vi "GEOM_File2keys.vi"(8 "error in (no error)":errorcluster, 10 "template in":string, 11 "ref dir":path) -> (0 "error out":errorcluster, 1 "header template":path, 2 "number of keywords found":i32, 3 "HeaderModules":T1[](array[typedef]))   [LabVIEW 2016]
doc: "This VI reads the configuration file searching for the \"infofile\" keyword. Then, it goes and reads the specified file, which should be a template for the TCS info format"
uses:
  GEOM_HeaderModule.ctl
panel:
  in  "HeaderModule":T1
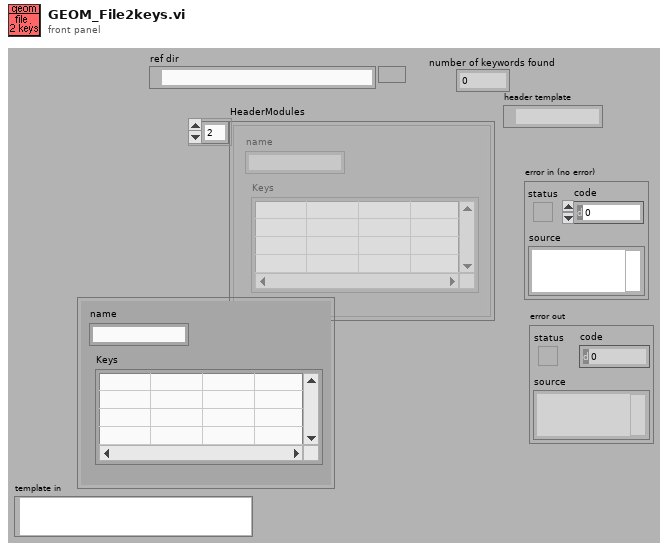
[diagram p1: front panel]
types:
  T1 = typedef "GEOM_HeaderModule.ctl" = cluster{"name":string, "Keys":string[][]}
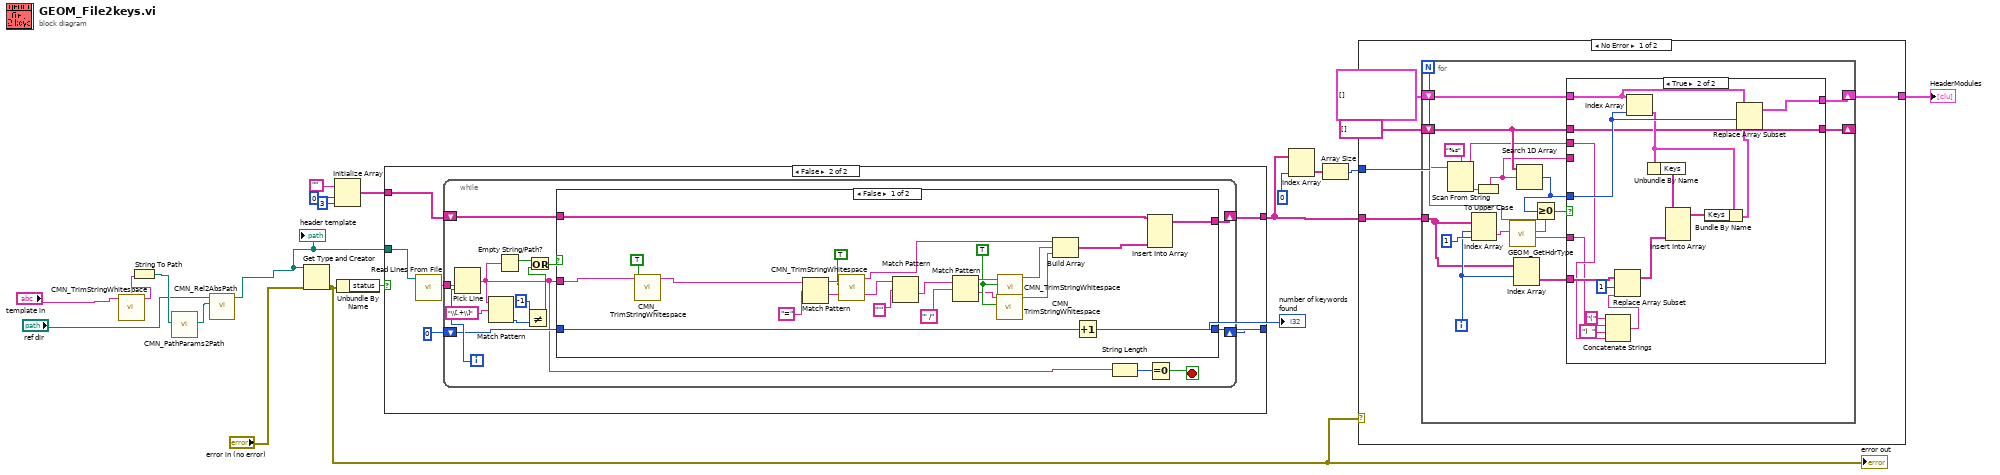
[diagram p0: block diagram]
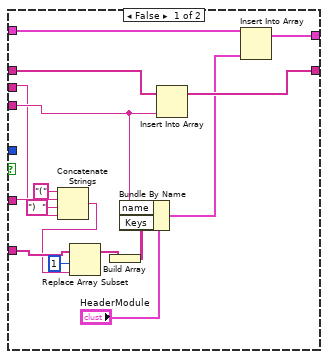
[diagram p2: hidden frame]
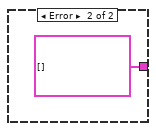
[diagram p3: hidden frame]
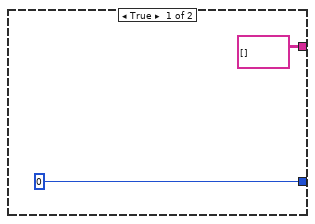
[diagram p4: hidden frame]
diagram:
  n1 = call "CMN_TrimStringWhitespace.vi"("string"="template in") -> ("trimmed string"=w5:string)  [unwired: 1 in, 8 out]
  n2 = String To Path(string=w5) -> (path=w4:path)
  n3 = call "CMN_PathParams2Path.vi"("Path In"=w4) -> ("Path out"=w3:path)  [unwired: 2 in, 8 out]
  n4 = call "CMN_Rel2AbsPath.vi"("test path"=w3, "absolute path"="ref dir") -> ("output path"=w13:path)  [unwired: 1 in, 8 out]
  "header template" <- w13
  n5 = Get Type and Creator(4:"error in (no error)", 7:w13) -> (0:w7:errorcluster)  [unwired: 3 out]
  "error out" <- w7
  n6 = Initialize Array("", 0, 3 ("dimension size")) -> (w15:string[][])
  n7 = Unbundle By Name(w7) -> ("status"=w18:bool)
  n8 = case shown="False" w18 {
    tunnel: w13 -> [_ w26]
    tunnel: [0 w23] -> w19
    tunnel: [string[][] [] w22] -> w11
    tunnel: w15 -> [_ w25]
    frame True {
    }
    frame False {
      n9 = call <vilib>:"Read Lines From File.vi"("file path (dialog if empty)"=w26) -> ("line string"=w27:string)  [unwired: 1 in, 7 out]
      n10 = while {
        shift-left: 0 -> [w32]
        shift-right: [w34] -> w23
        shift-left: w25 -> [w39]
        shift-right: [w38] -> w22
        tunnel: w27 -> [w42]
        i -> [w33]
        stop <- w40 stop-if-true
        n11 = Pick Line(multi-line string=w42, line index=w33) -> (output string=w29:string)  [unwired: 1 out]
        n12 = Match Pattern(string=w29, regular expression="\\[.+\\]") -> (offset past match=w36:i32)  [unwired: 4 out]
        n13 = Empty String/Path?(string/path=w29) -> (empty?=w31:bool)
        n14 = Not Equal?(x=-1, y=w36) -> (x != y?=w30:bool)
        n15 = Or(x=w31, y=w30) -> (x .or. y?=w28:bool)
        n16 = case shown="False" w28 {
          tunnel: w32 -> [w46 w64]
          tunnel: w39 -> [w50 w65]
          tunnel: [w49 w65] -> w38
          tunnel: [w45 w64] -> w34
          tunnel: w29 -> [w44 _]
          frame False {
            w55 = TRUE ("Both Ends?(F)")
            n17 = call "CMN_TrimStringWhitespace.vi"("Both Ends?(T)"=TRUE ("Both Ends?(F)"), "string"=w44) -> ("trimmed string"=w43:string)  [unwired: 8 out]
            n18 = Match Pattern(string=w43, regular expression="=") -> (before substring=w62:string, after substring=w61:string)  [unwired: 3 out]
            n19 = call "CMN_TrimStringWhitespace.vi"("Both Ends?(T)"=TRUE ("Both Ends?(F)"), "string"=w62) -> ("trimmed string"=w47:string)  [unwired: 8 out]
            n20 = Match Pattern(string=w61, regular expression="'") -> (after substring=w59:string)  [unwired: 4 out]
            n21 = Match Pattern(string=w59, regular expression="' /") -> (before substring=w57:string, after substring=w54:string)  [unwired: 3 out]
            n22 = call "CMN_TrimStringWhitespace.vi"("Both Ends?(T)"=w55, "string"=w54) -> ("trimmed string"=w52:string)  [unwired: 8 out]
            n23 = call "CMN_TrimStringWhitespace.vi"("Both Ends?(T)"=w55, "string"=w57) -> ("trimmed string"=w53:string)  [unwired: 8 out]
            n24 = Build Array(w47, w53, w52) -> (w51:string[])
            n25 = Increment(x=w46) -> (x+1=w45:i32)
            n26 = Insert Into Array(array=w50, new element=w51) -> (w49:string[][])  [unwired: 2 in]
          }
          frame True {
          }
        }
        n27 = String Length(string=w29) -> (length=w41:i32)
        n28 = Equal To 0?(x=w41) -> (x = 0?=w40:bool)
      }
    }
  }
  "number of keywords found" <- w19
  n29 = Index Array(array=w11, index (col)=0 ("disabled index (col)")) -> (element=w9:string[])  [unwired: 1 in]
  n30 = Array Size(array=w9) -> (size(s)=w8:i32)
  n31 = case shown="No Error" w7 {
    tunnel: w11 -> [w70 _]
    tunnel: w8 -> [w69 _]
    tunnel: [w66 T1[] []] -> w6
    frame No Error {
      n32 = for {
        N: w69 -> [_]
        tunnel: w70 -> [w76]
        shift-right: [w83] -> _
        shift-left: string[] [] -> [w81]
        shift-right: [w79] -> w66
        shift-left: T1[] [] -> [w78]
        i -> [w77]
        n33 = Index Array(array=w76, index (row)=w77, index (col)=1 ("disabled index (col)")) -> (element=w73:string)
        n34 = call "GEOM_GetHdrType.vi"("arg in"=w73) -> ("type"=w71:string, "arg out"=w72:string)  [unwired: 9 out]
        n35 = Scan From String(format string="%s", input string=w72) -> (remaining string=w80:string, output 1=w84:string)  [unwired: 2 in, 3 out]
        n36 = To Upper Case(1:w84) -> (0:w74:string)
        n37 = Index Array(array=w76, index (row)=w77) -> (element=w75:string[])  [unwired: 1 in]
        n38 = Search 1D Array(1D array=w81, element=w74) -> (index of element=w82:i32)  [unwired: 1 out]
        n39 = Greater Or Equal To 0?(x=w82) -> (x >= 0?=w85:bool)
        n40 = case shown="True" w85 {
          tunnel: w74 -> [w100 _]
          tunnel: [w103 w112] -> w83
          tunnel: w82 -> [_ w118]
          tunnel: w81 -> [w102 w112]
          tunnel: w80 -> [w90 w106]
          tunnel: [w97 w119] -> w79
          tunnel: w78 -> [w96 w113]
          tunnel: w75 -> [w94 w111]
          tunnel: w71 -> [w92 w105]
          frame False {
            n41 = Concatenate Strings("(" ("string"), w92, ")  " ("string"), w90) -> (w91:string)
            n42 = Replace Array Subset(array=w94, new element=w91, index=1) -> (w93:string[])
            n43 = Build Array(w93) -> (w99:string[][])
            n44 = Bundle By Name(cluster="HeaderModule", "name"=w100, "Keys"=w99) -> (w98:T1)
            n45 = Insert Into Array(array=w102, new element=w100) -> (w103:string[])  [unwired: 1 in]
            n46 = Insert Into Array(array=w96, new element=w98) -> (w97:T1[])  [unwired: 1 in]
          }
          frame True {
            n47 = Concatenate Strings("(" ("string"), w105, ")  " ("string"), w106) -> (w104:string)
            n48 = Replace Array Subset(array=w111, new element=w104, index=1) -> (w110:string[])
            n49 = Index Array(array=w113, index=w118) -> (element=w115:T1)
            n50 = Unbundle By Name(w115) -> ("Keys"=w117:string[][])
            n51 = Insert Into Array(array=w117, new element=w110) -> (w116:string[][])  [unwired: 2 in]
            n52 = Bundle By Name(cluster=w115, "Keys"=w116) -> (w114:T1)
            n53 = Replace Array Subset(array=w113, new element=w114, index=w118) -> (w119:T1[])
          }
        }
      }
    }
    frame Error {
    }
  }
  "HeaderModules" <- w6
